vi "processGetStopMech.vi"(6 "stopMechanismType":T1, 8 "error in (no error)":errorcluster, 11 "targetClassPath":path) -> (0 "error out":errorcluster)   [LabVIEW 2023]
uses:
  stopMechanismType.ctl
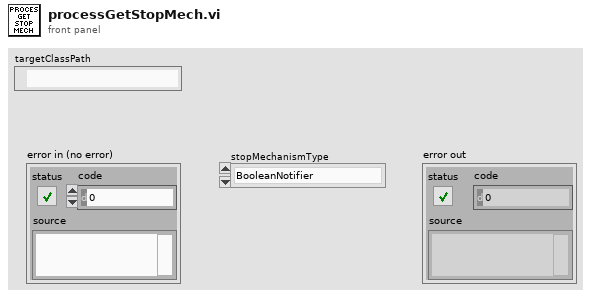
[diagram p1: front panel]
types:
  T1 = typedef "stopMechanismType.ctl" = enum16{"BooleanNotifier", "BooleanUE", "MsgUE"}
  T2 = cluster{"placeholderName":string, "methodName":string}
  T3 = cluster{"placeholderName":string, "methodName":string}[]
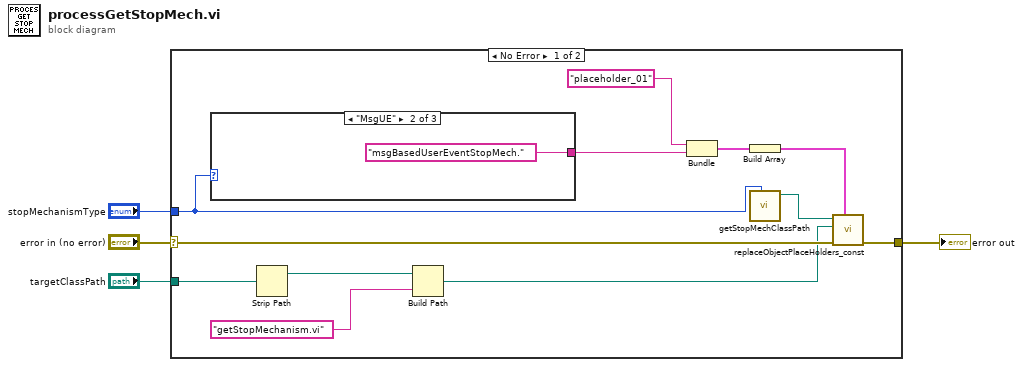
[diagram p0: block diagram]
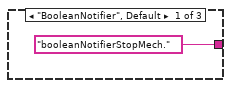
[diagram p2: hidden frame]
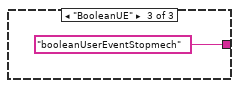
[diagram p3: hidden frame]
diagram:
  n1 = case shown="No Error" "error in (no error)" {
    selector: "error in (no error)" -> [w16 w20]
    tunnel: [w15 w20] -> w3
    tunnel: "stopMechanismType" -> [w10 _]
    tunnel: "targetClassPath" -> [w8 _]
    frame No Error {
      n2 = case shown="\"MsgUE\"" w10 {
        tunnel: ["booleanNotifierStopMech." ("methodName") "msgBasedUserEventStopMech." ("methodName") "booleanUserEventStopmech" ("methodName")] -> w14
        frame "BooleanNotifier", Default {
        }
        frame "MsgUE" {
        }
        frame "BooleanUE" {
        }
      }
      n3 = Strip Path(path=w8) -> (stripped path=w7:path)  [unwired: 1 out]
      n4 = Build Path(base path=w7, name or relative path="getStopMechanism.vi" ("methodName")) -> (appended path=w5:path)
      n5 = Bundle("placeholderName"="placeholder_01", "methodName"=w14) -> (w12:T2)  [unwired: 1 in]
      n6 = Build Array(w12) -> (w11:T3)
      n7 = call "getStopMechClassPath.vi"("stopMechanismType"=w10) -> ("ITaskClassPath"=w9:path)  [unwired: 8 in]
      n8 = call "replaceObjectPlaceHolders_const.vi"("placeholderList"=w11, "error in (no error)"=w16, "targetVI"=w5, "classPathToReplace"=w9) -> ("error out"=w15:errorcluster)  [unwired: 7 in]
    }
    frame Error {
    }
  }
  "error out" <- w3
